vi "calc_singleManipJumpWaveform_v0.02.vi"(0 "New input cluster":T1={"Start Position (N)"=enum."Jumper Safe Position", "Duration (s)"=8.0, "Delay (s)"=0.5, "Pulse Width (s)"=0.0, "Valve 1 Position"=0, "Valve 2 Position"=0, "Replicates"=0.0, "Jump Position (m)"=enum."Jumper Safe Position", "Vholding (mV)"=0.0, "Valve 3 Position"=0, "valve 1 used now?"=TRUE, "valve 2 used now?"=FALSE, "valve 3 used now? "=FALSE, "protocol Preview"=[]}, 1 "Clear Waveform?":bool, 5 "Old input cluster":T1={"Start Position (N)"=enum."Jumper Safe Position", "Duration (s)"=8.0, "Delay (s)"=0.5, "Pulse Width (s)"=0.0, "Valve 1 Position"=0, "Valve 2 Position"=0, "Replicates"=0.0, "Jump Position (m)"=enum."Jumper Safe Position", "Vholding (mV)"=0.0, "Valve 3 Position"=0, "valve 1 used now?"=TRUE, "valve 2 used now?"=FALSE, "valve 3 used now? "=FALSE, "protocol Preview"=[]}, 7 "simulate Wave freq":i32=10000, 11 "error in":errorcluster) -> (4 "output cluster":T1={"Start Position (N)"=enum."Jumper Safe Position", "Duration (s)"=8.0, "Delay (s)"=0.5, "Pulse Width (s)"=0.0, "Valve 1 Position"=0, "Valve 2 Position"=0, "Replicates"=0.0, "Jump Position (m)"=enum."Jumper Safe Position", "Vholding (mV)"=0.0, "Valve 3 Position"=0, "valve 1 used now?"=TRUE, "valve 2 used now?"=FALSE, "valve 3 used now? "=FALSE, "protocol Preview"=[]}, 15 "error out":errorcluster)   [LabVIEW 2019]
uses:
  <vilib>/measure/NI_MABase.lvlib
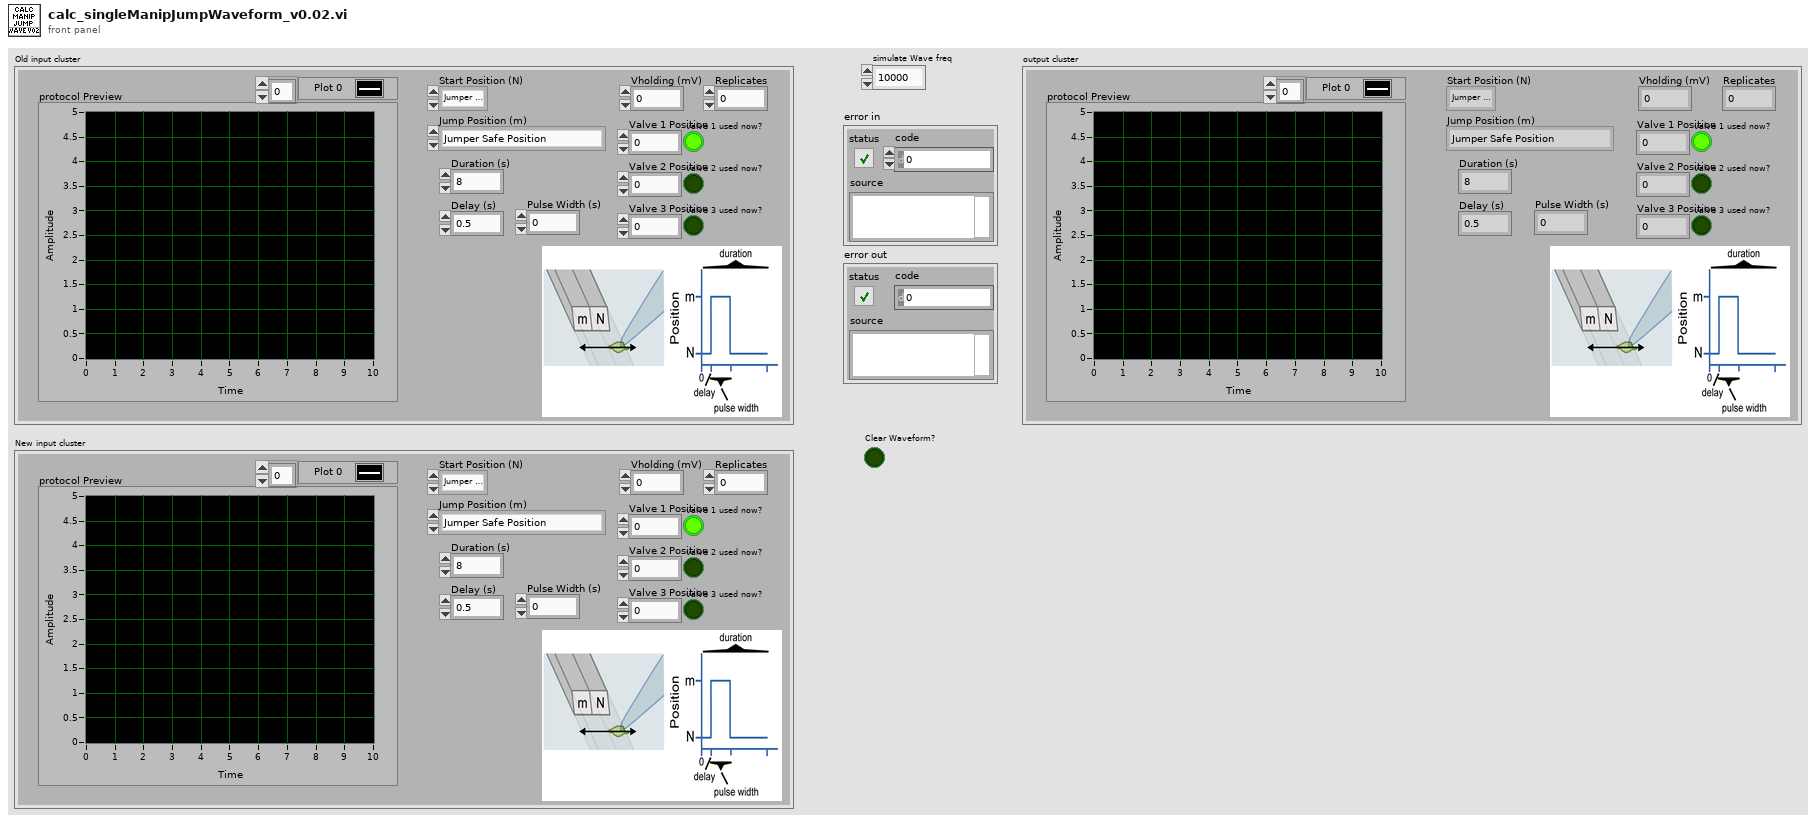
[diagram p1: front panel]
types:
  T1 = cluster{"Start Position (N)":enum16{"Jumper Safe Position", "Experiment Safe Position", "Jumper Position A", "Jumper Position B", "Jumper Position C", "Jumper Position o-A", "Jumper Position A-o", "Jumper Position A-B", "Jumper Position B-A", "Jumper Position B-C", "Jumper Position C-B", "Jumper Position C-o", "Jumper Position o-C", "Don't Move"}, "Duration (s)":dbl, "Delay (s)":dbl, "Pulse Width (s)":dbl, "Valve 1 Position":i16, "Valve 2 Position":i16, "Replicates":dbl, "Jump Position (m)":enum16{"Jumper Safe Position", "Experiment Safe Position", "Jumper Position A", "Jumper Position B", "Jumper Position C", "Jumper Position o-A", "Jumper Position A-o", "Jumper Position A-B", "Jumper Position B-A", "Jumper Position B-C", "Jumper Position C-B", "Jumper Position C-o", "Jumper Position o-C", "Don't Move"}, "Vholding (mV)":dbl, "Valve 3 Position":i16, "valve 1 used now?":bool, "valve 2 used now?":bool, "valve 3 used now? ":bool, "protocol Preview":waveform(dbl)[]}
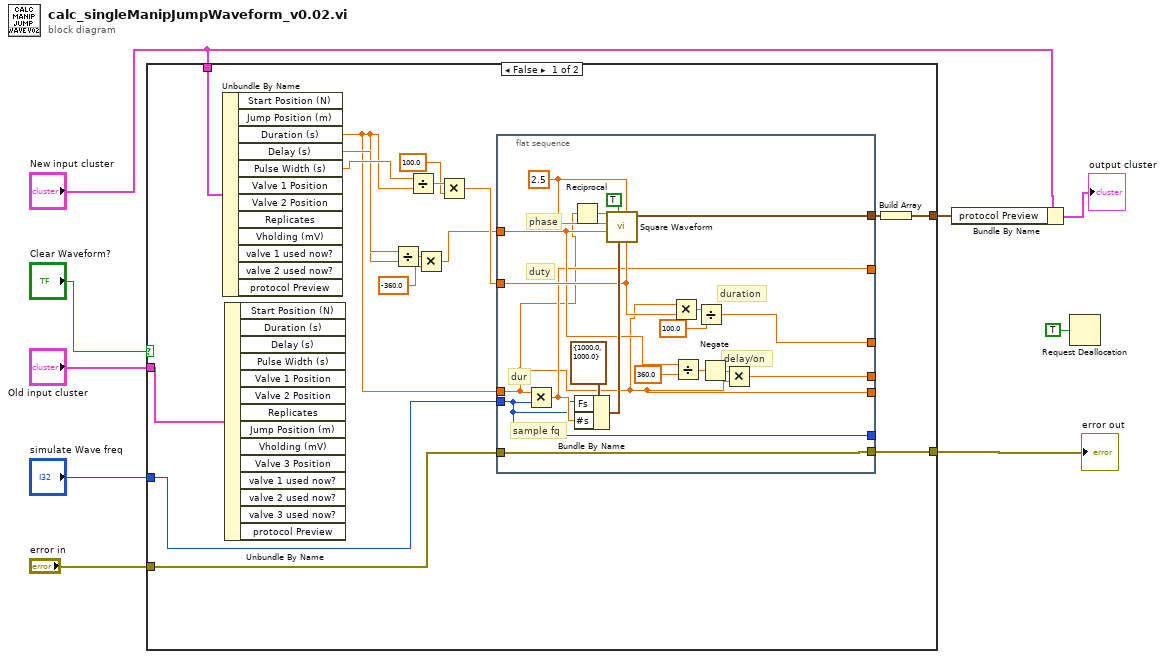
[diagram p0: block diagram]
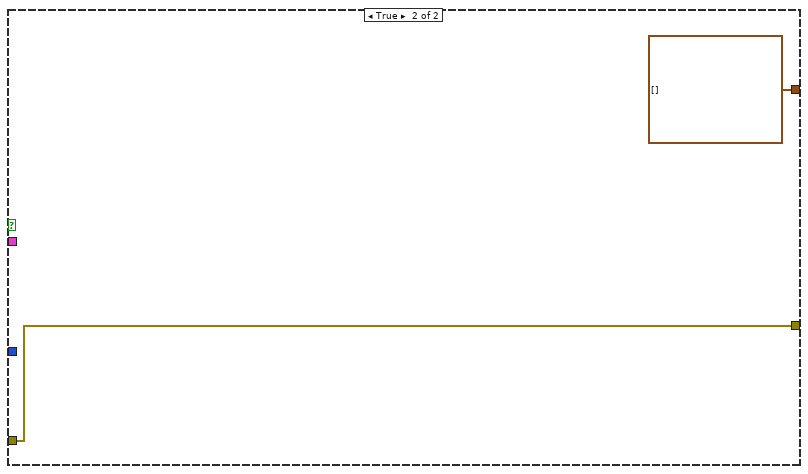
[diagram p2: hidden frame]
diagram:
  n1 = case shown="False" "Clear Waveform?" {
    tunnel: "error in" -> [w16 w45]
    tunnel: "New input cluster" -> [w15 _]
    tunnel: [w13 waveform(dbl)[] []] -> w6
    tunnel: [w12 w45] -> w5
    tunnel: "simulate Wave freq" -> [w11 _]
    tunnel: "Old input cluster" -> [w10 _]
    frame False {
      n2 = Unbundle By Name(w15) -> ("Duration (s)"=w19:dbl, "Delay (s)"=w24:dbl, "Pulse Width (s)"=w25:dbl)  [unwired: 9 out]
      n3 = Unbundle By Name(w10) -> ()  [unwired: 14 out]
      n4 = Divide(x=w24, y=w19) -> (x/y=w20:dbl)
      n5 = Divide(x=w25, y=w19) -> (x/y=w23:dbl)
      n6 = Multiply(x=w20, y=-360.0) -> (x*y=w17:dbl)
      n7 = Multiply(x=w23, y=100.0) -> (x*y=w18:dbl)
      n8 = flat-sequence {
        tunnel: w17 -> [w37]
        tunnel: w18 -> [w40]
        tunnel: w19 -> [w28]
        tunnel: w11 -> [w27]
        tunnel: w16 -> [w26]
        tunnel: [w32] -> w14
        tunnel: [w31] -> _
        tunnel: [w30] -> _
        tunnel: [w29] -> _
        tunnel: [w28] -> _
        tunnel: [w27] -> _
        tunnel: [w26] -> w12
        frame #0 {
          w44 = 2.5 ("Amplitude")
          # "sample fq"
          # "dur"
          # "duty"
          # "phase"
          # "delay/on"
          # "duration"
          n9 = Multiply(x=w28, y=w27) -> (x*y=w31:dbl)
          n10 = Reciprocal(x=w28) -> (1/x=w33:dbl)
          n11 = Bundle By Name(cluster=cluster{"Fs":dbl, "#s":dbl} {"Fs"=1000.0, "#s"=1000.0} ("sampling info"), "Fs"=w27, "#s"=w31) -> (w41:cluster{"Fs":dbl, "#s":dbl})
          n12 = call <vilib>:"Square Waveform.vi"("duty cycle (%)"=w40, "offset"=w44, "sampling info"=w41, "reset signal"=TRUE, "phase"=w37, "amplitude"=w44, "frequency"=w33) -> ("signal out"=w32:waveform(dbl))  [unwired: 3 in, 1 out]
          n13 = Multiply(x=w28, y=w40) -> (x*y=w39:dbl)
          n14 = Divide(x=w37, y=360.0) -> (x/y=w35:dbl)
          n15 = Divide(x=w39, y=100.0) -> (x/y=w30:dbl)
          n16 = Negate(x=w35) -> (-x=w34:dbl)
          n17 = Multiply(x=w34, y=w28) -> (x*y=w29:dbl)
        }
      }
      n18 = Build Array(w14) -> (w13:waveform(dbl)[])
    }
    frame True {
    }
  }
  "error out" <- w5
  n19 = Bundle By Name(cluster="New input cluster", "protocol Preview"=w6) -> (→"output cluster":T1)
  n20 = Request Deallocation(TRUE ("flag")) -> ()
